vi "sensor array.vi"() -> ()   [LabVIEW 2018]
uses:
  <vilib>/Waveform/WDTOps.llb/WDT Get Waveform Time Array DBL.vi
panel:
  out "sensor":cluster{"Y":dbl[], "Y":dbl[]}[](graph)
  out "heat":cluster{"Y":dbl[], "Y":dbl[]}[](graph)
  in  "停止":bool
  out "source":string
  in  "File Path":path
  in  "File Name":string
  out "sensor4":dynamicdata(graph)
  out "sensor3":dynamicdata(graph)
  out "sensor2":dynamicdata(graph)
  out "sensor1":dynamicdata(graph)
  in  "设备名":tag="Dev1"
  in  "速率":dbl=1000.0
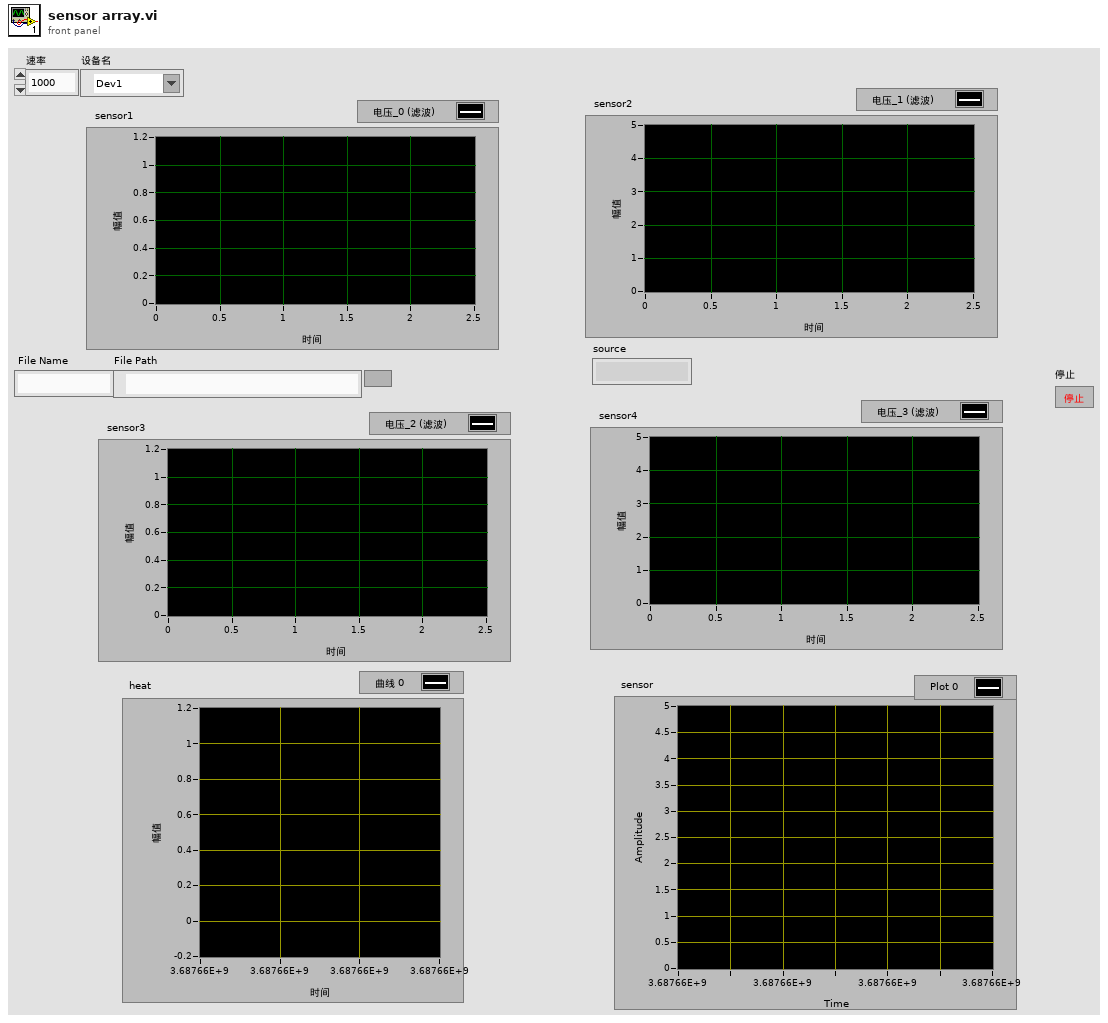
[diagram p1: front panel]
types:
  T1 = enum16{"open", "replace", "create", "open or create", "replace or create", "replace or create with confirmation"}
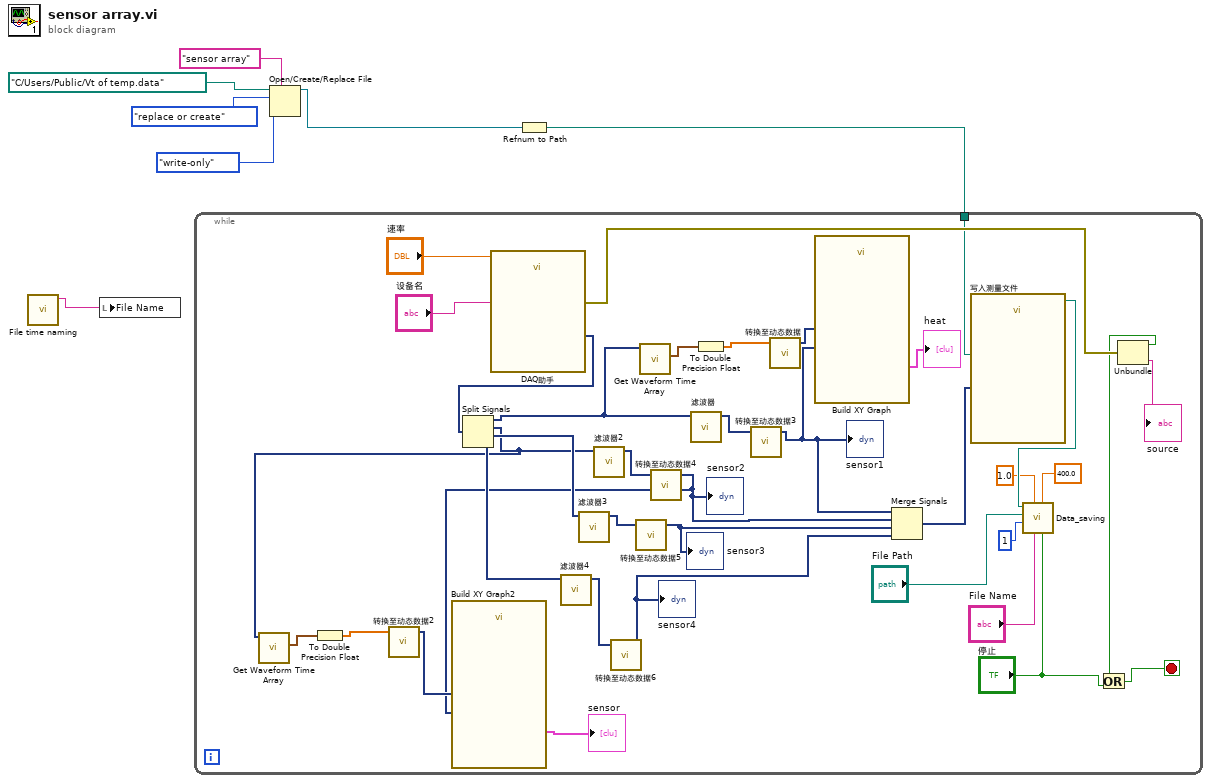
[diagram p0: block diagram]
diagram:
  n1 = call "File time naming.vi"() -> ("result string"=w1:string)  [unwired: 11 in]
  n2 = local write "File Name"(w1) -> ()
  n3 = Open/Create/Replace File(file path (use dialog)=path "C:/Users/Public/Vt of temp.data" ("文件路径（使用对话框）"), prompt="sensor array" ("提示"), operation (0:open)=T1."replace or create" ("操作(0:open)"), access (0:read/write)=enum16{"read/write", "read-only", "write-only"}."write-only" ("权限(0:read/write)")) -> (refnum out=w3:refnum<file>)  [unwired: 2 in, 2 out]
  n4 = Refnum to Path(1:w3) -> (0:w2:path)
  n5 = while {
    tunnel: w2 -> [w36]
    stop <- w26 stop-if-true
    n6 = call "DAQ助手"("速率"="速率", "设备名"="设备名") -> ("data"=w41:dynamicdata, "error out"=w37:errorcluster)  [unwired: 14 in, 2 out]
    n7 = Split Signals(w41) -> (w25:dynamicdata, w17:dynamicdata, w40:dynamicdata, w39:dynamicdata)  [unwired: 4 in]
    n8 = call-poly <vilib>:"Get Waveform Time Array.vi"("waveform in"=w17) -> ("X array"=w20:timestamp[])  [unwired: 9 in, 1 out]
    n9 = To Double Precision Float(number=w20) -> (double precision float=w19:dbl[])
    n10 = call "转换至动态数据2"("Array"=w19) -> ("Dynamic Data Type"=w18:dynamicdata)  [unwired: 3 in]
    n11 = call "滤波器4"("Signal"=w39) -> ("Filtered Signal"=w10:dynamicdata)  [unwired: 9 in, 1 out]
    n12 = call "滤波器3"("Signal"=w40) -> ("Filtered Signal"=w12:dynamicdata)  [unwired: 9 in, 1 out]
    n13 = call "滤波器2"("Signal"=w17) -> ("Filtered Signal"=w13:dynamicdata)  [unwired: 9 in, 1 out]
    n14 = call "转换至动态数据6"("Waveform"=w10) -> ("Dynamic Data Type"=w9:dynamicdata)  [unwired: 3 in]
    "sensor4" <- w9
    n15 = call "转换至动态数据5"("Waveform"=w12) -> ("Dynamic Data Type"=w11:dynamicdata)  [unwired: 3 in]
    "sensor3" <- w11
    n16 = call-poly <vilib>:"Get Waveform Time Array.vi"("waveform in"=w25) -> ("X array"=w24:timestamp[])  [unwired: 9 in, 1 out]
    n17 = call "转换至动态数据4"("Waveform"=w13) -> ("Dynamic Data Type"=w8:dynamicdata)  [unwired: 3 in]
    "sensor2" <- w8
    n18 = call "Build XY Graph2"("Y Input"=w8, "X Input"=w18) -> ("XY Graph"=→"sensor":cluster{"Y":dbl[], "Y":dbl[]}[])  [unwired: 3 in, 6 out]
    n19 = call "滤波器"("Signal"=w25) -> ("Filtered Signal"=w15:dynamicdata)  [unwired: 9 in, 1 out]
    n20 = To Double Precision Float(number=w24) -> (double precision float=w23:dbl[])
    n21 = call "转换至动态数据3"("Waveform"=w15) -> ("Dynamic Data Type"=w14:dynamicdata)  [unwired: 3 in]
    "sensor1" <- w14
    n22 = call "转换至动态数据"("Array"=w23) -> ("Dynamic Data Type"=w22:dynamicdata)  [unwired: 3 in]
    n23 = call "Build XY Graph"("Y Input"=w14, "X Input"=w22) -> ("XY Graph"=→"heat":cluster{"Y":dbl[], "Y":dbl[]}[])  [unwired: 3 in, 6 out]
    n24 = Merge Signals(w14, w8, w11, w9) -> (w38:dynamicdata)
    n25 = call "写入测量文件"("Signals"=w38, "Filename"=w36) -> ("Filename Out"=w32:path)  [unwired: 15 in, 2 out]
    n26 = call "Data_saving.vi"("Boolean"="停止", "Sampling Rate"=400.0, "File Name"="File Name", "Voltage Sensitivity\n1000 will be 1000"=1.0 ("Voltage Sensitivity\n1000 will be 1000"), "Number of Samples Per Channel"=1, "File Path"="File Path", "File name source"=w32) -> ()  [unwired: 5 in]
    n27 = Unbundle(w37) -> ("status"=w27:bool, "source"=→"source":string)  [unwired: 1 out]
    n28 = Or(x=w27, y="停止") -> (x .or. y?=w26:bool)
  }
